vi "ecg_ncs_v4.vi"() -> ()   [LabVIEW 2016]
uses:
  <instrlib>/niUSRP/niUSRP Timestamp.ctl
  C:/Program Files/National Instruments/LabVIEW 2016/examples/Instrument IO/Serial/support/Serial - Settings.ctl
  State.ctl
  <vilib>/Instr/_visa.llb/VISA Configure Serial Port (Instr).vi
  <instrlib>/niUSRP/niUSRP Write Tx Data (2D CDB).vi
  <instrlib>/niUSRP/niUSRP Fetch Rx Data (2D CDB).vi
panel:
  in  "File Name 2":string="Test"
  in  "Path 2":path=path "D:/Research/SummerFall17Spring18/CnC/NCS/EcgNcsCorrelation/Labview Codes/ECG_NCS"
  out "#Loop = #Packets Received":i32
  out "ECGsample":i16
  out "PhNcs":dbl
  out "AmpNcs":dbl
  out "AmpNcsDS":dbl
  out "PhNcsDS":dbl
  out "error IO 2":errorcluster={"status"=FALSE, "code"=-1074118647, "source"=""}
  in  "Serial Settings":T1={"baud rate"=57600, "data bits"=8, "parity"=enum."None", "stop bits"=10, "flow control"=0} {"flow control" items=["None"=0, "XON/XOFF"=1, "RTS/CTS"=2, "DTR/DSR"=4]; "stop bits" items=["1.0"=10, "1.5"=15, "2.0"=20]; "data bits" min=5 max=8 step=1; "baud rate" items=["75"=75, "110"=110, "134"=134, "150"=150, "300"=300, "600"=600, "1200"=1200, "1800"=1800, "2400"=2400, "4800"=4800, "7200"=7200, "9600"=9600, "14400"=14400, "19200"=19200, "28800"=28800, "38400"=38400, "56000"=56000, "57600"=57600, "115200"=115200, "128000"=128000, "230400"=230400]}
  in  "VISA resource name":refnum<visa-resource-name>="bmd101"
  out "ECG":i16(graph)
  in  "byte count":u32=1
  out "Coerced Rx IQ Rate":dbl
  in  "Sampling Rate":i32=500
  out "Gain":dbl=-15.0
  out "Bandwidth":dbl=56000000.0
  out "Coerced Carrier Frequency":dbl=2000000000.0 format="%#.17g"
  out "Coerced Tx IQ rate":dbl=1000000.0
  out "error IO":errorcluster={"status"=FALSE, "code"=-1074118647, "source"=""}
  in  "Rx Number of Samples":i32=10000
  in  "Tab Control 2":enum32{"NI-294x/295x", "NI-2900/2901"}(tab)=enum."NI-2900/2901"
  in  "Rx carrier frequency [Hz]":dbl=2000000000.0 format="%#_6p"
  in  "Tx carrier frequency [Hz]":dbl=1000000000.0 format="%#_6p"
  in  "Start Trigger Time":T2={"whole seconds"=1, "fractional seconds"=0.0}
  in  "Tab Control":T3(tab)
  out "NCS tag Amp":dbl[](graph)=[0.011967714738528729, 0.012021355192189592, 0.012015275039596582, 0.011969166030167903, 0.011958890166168242, 0.012007893820858737, 0.012022893722444085, 0.011978222225113794, 0.011969989939463181, 0.012003099640895068]
  out "NCS tag Phase":dbl[](graph)=[0.011967714738528729, 0.012021355192189592, 0.012015275039596582, 0.011969166030167903, 0.011958890166168242, 0.012007893820858737, 0.012022893722444085, 0.011978222225113794, 0.011969989939463181, 0.012003099640895068]
  out "Tag Amp":dbl[](graph)
  out "Tag Phase":dbl[](graph)
  out "Tx Waveform Graph":waveform(dbl)[](graph)
  in  "Stop":bool
  in  "Channel 0\nTone Amplitude":dbl=0.707 step=0.05 format="%#.6g"
  in  "Channel 0 \nTone Frequency":dbl=5000.0 format="%#_6p"
  in  "Tx Waveform Size":dbl=2000.0
  in  "Device Name":refnum<k15>="MyB200"
  in  "Tx Gain":dbl=28.0 format="%#_6f"
  in  "Tx IQ Rate":dbl=1000000.0 format="%#_6p"
  in  "Rx Gain":dbl=32.0 format="%#_6f"
  in  "Rx IQ Rate":dbl=1000000.0 format="%#_6p"
  # "Rx Settings"
  # "Tx Settings"
  # "Note that on the NI-2900 and NI-2901, both Rx channels share an LO and both Tx channels share an LO. However, on the NI-294x/295x devices, Rx and Tx of channel 0 share an LO and Rx and Tx of channel 1 share an LO."
  # "Rx: Number of samples should be 1e6/512 in one loop."
  # "This Tx graph should always have end and start tied up since this is being sent in a loop continuously. Otherwise phase jumps will be noticed."
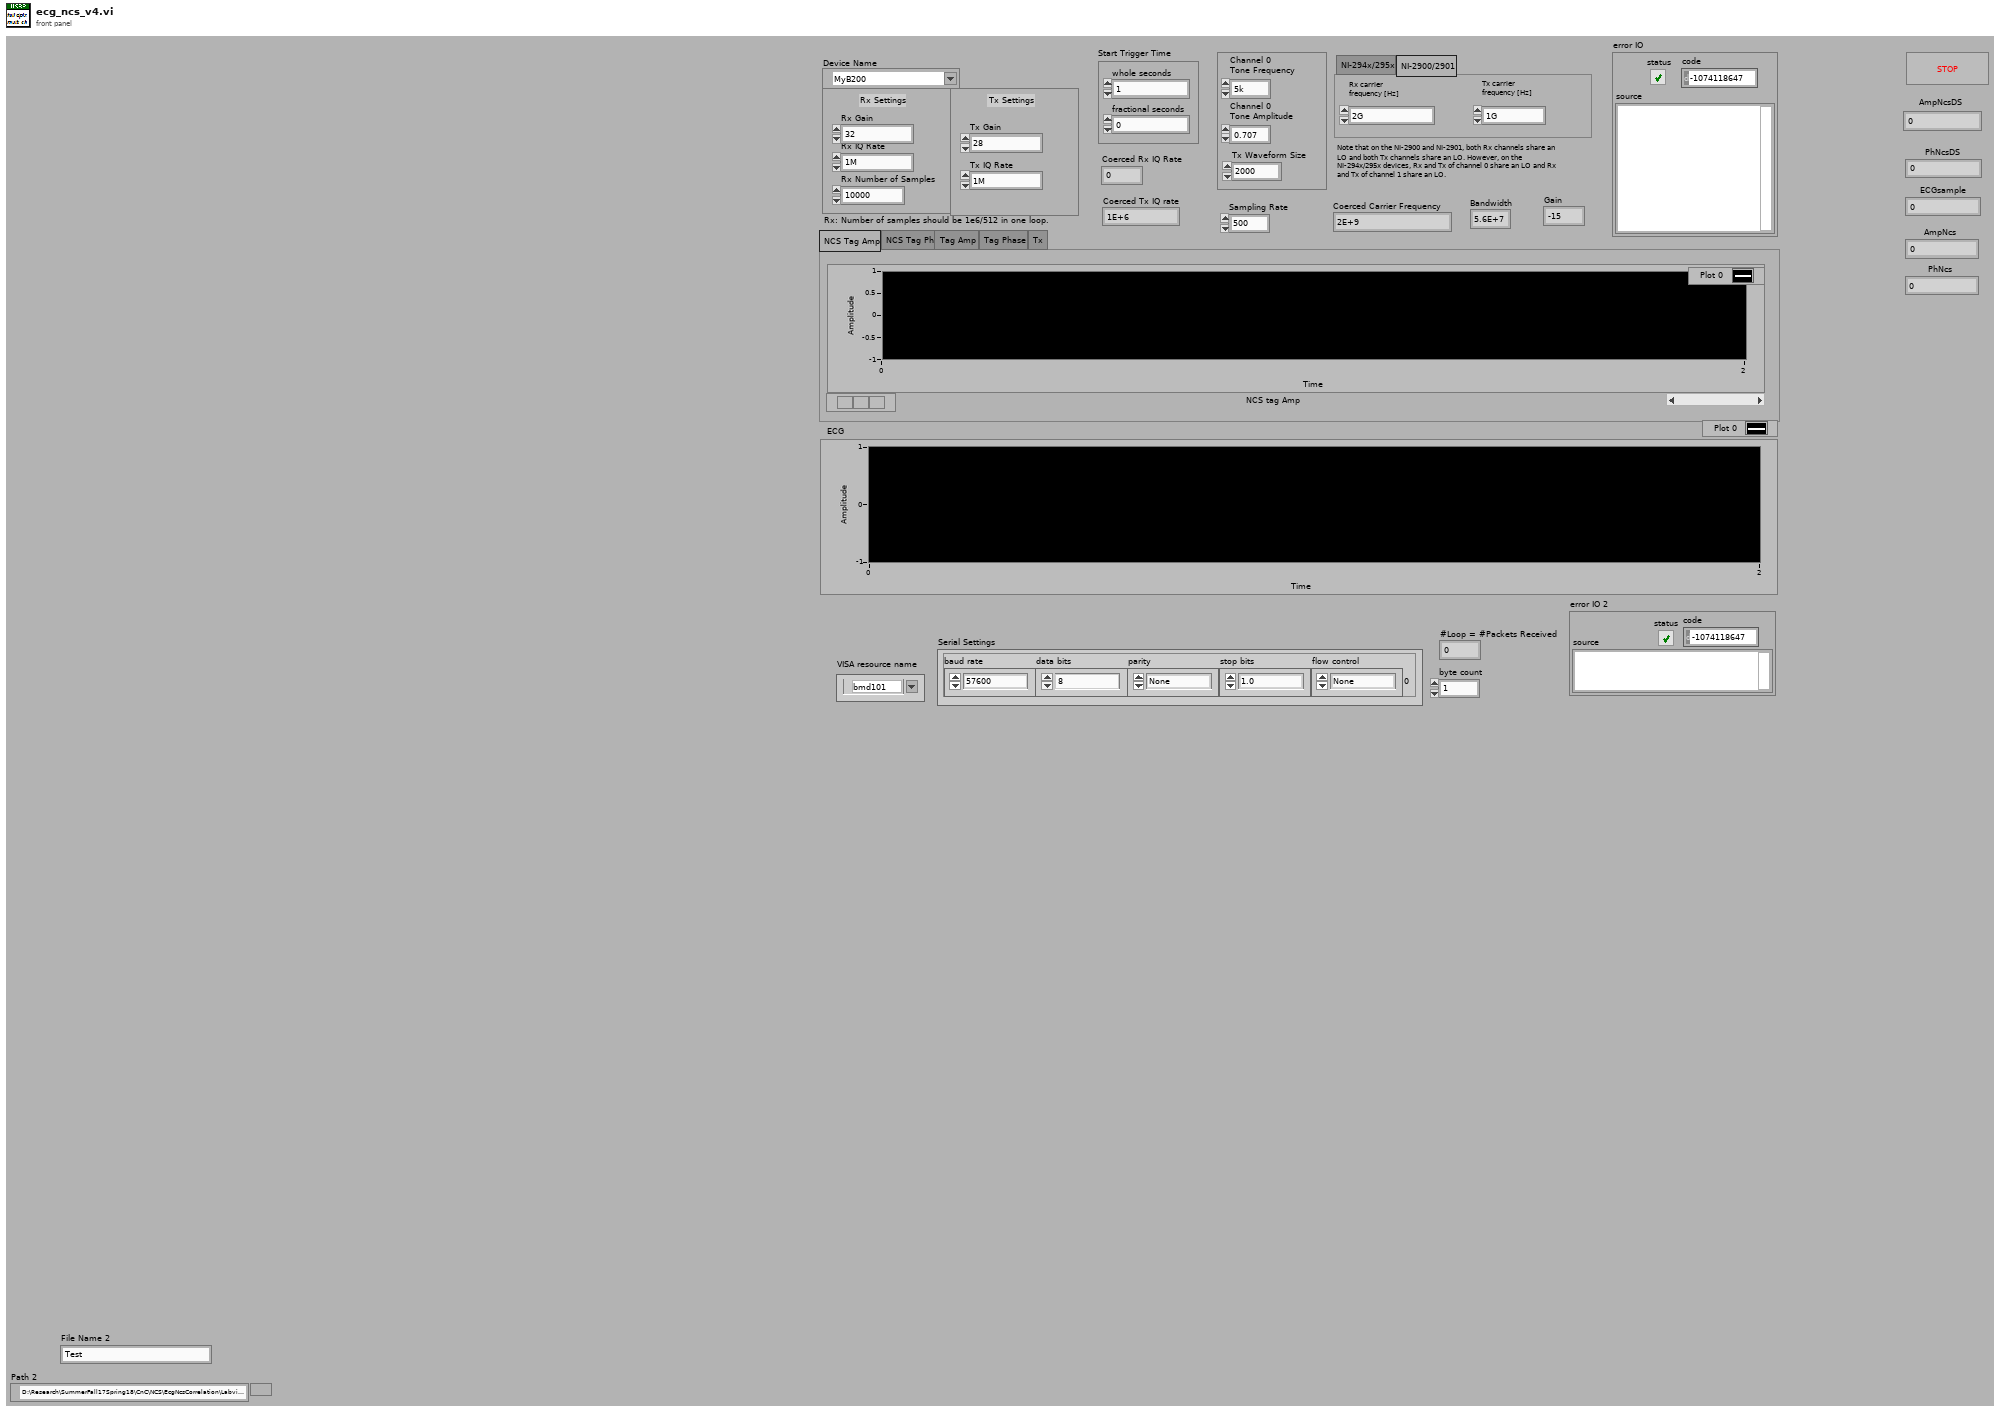
[diagram p1: front panel]
types:
  T1 = typedef "Serial - Settings.ctl" = cluster{"baud rate":u32, "data bits":u16, "parity":enum16{"None", "Odd", "Even", "Mark", "Space"}, "stop bits":u16, "flow control":u16}
  T2 = typedef "niUSRP Timestamp.ctl" = cluster{"whole seconds":u64, "fractional seconds":dbl}
  T3 = enum32{"NCS Tag Amp", "NCS Tag Ph", "Tag Amp", "Tag Phase", "Tx"}
  T4 = typedef "State.ctl" = enum16{"Initialize", "get byte", "check", "packet received", "packet approved"}
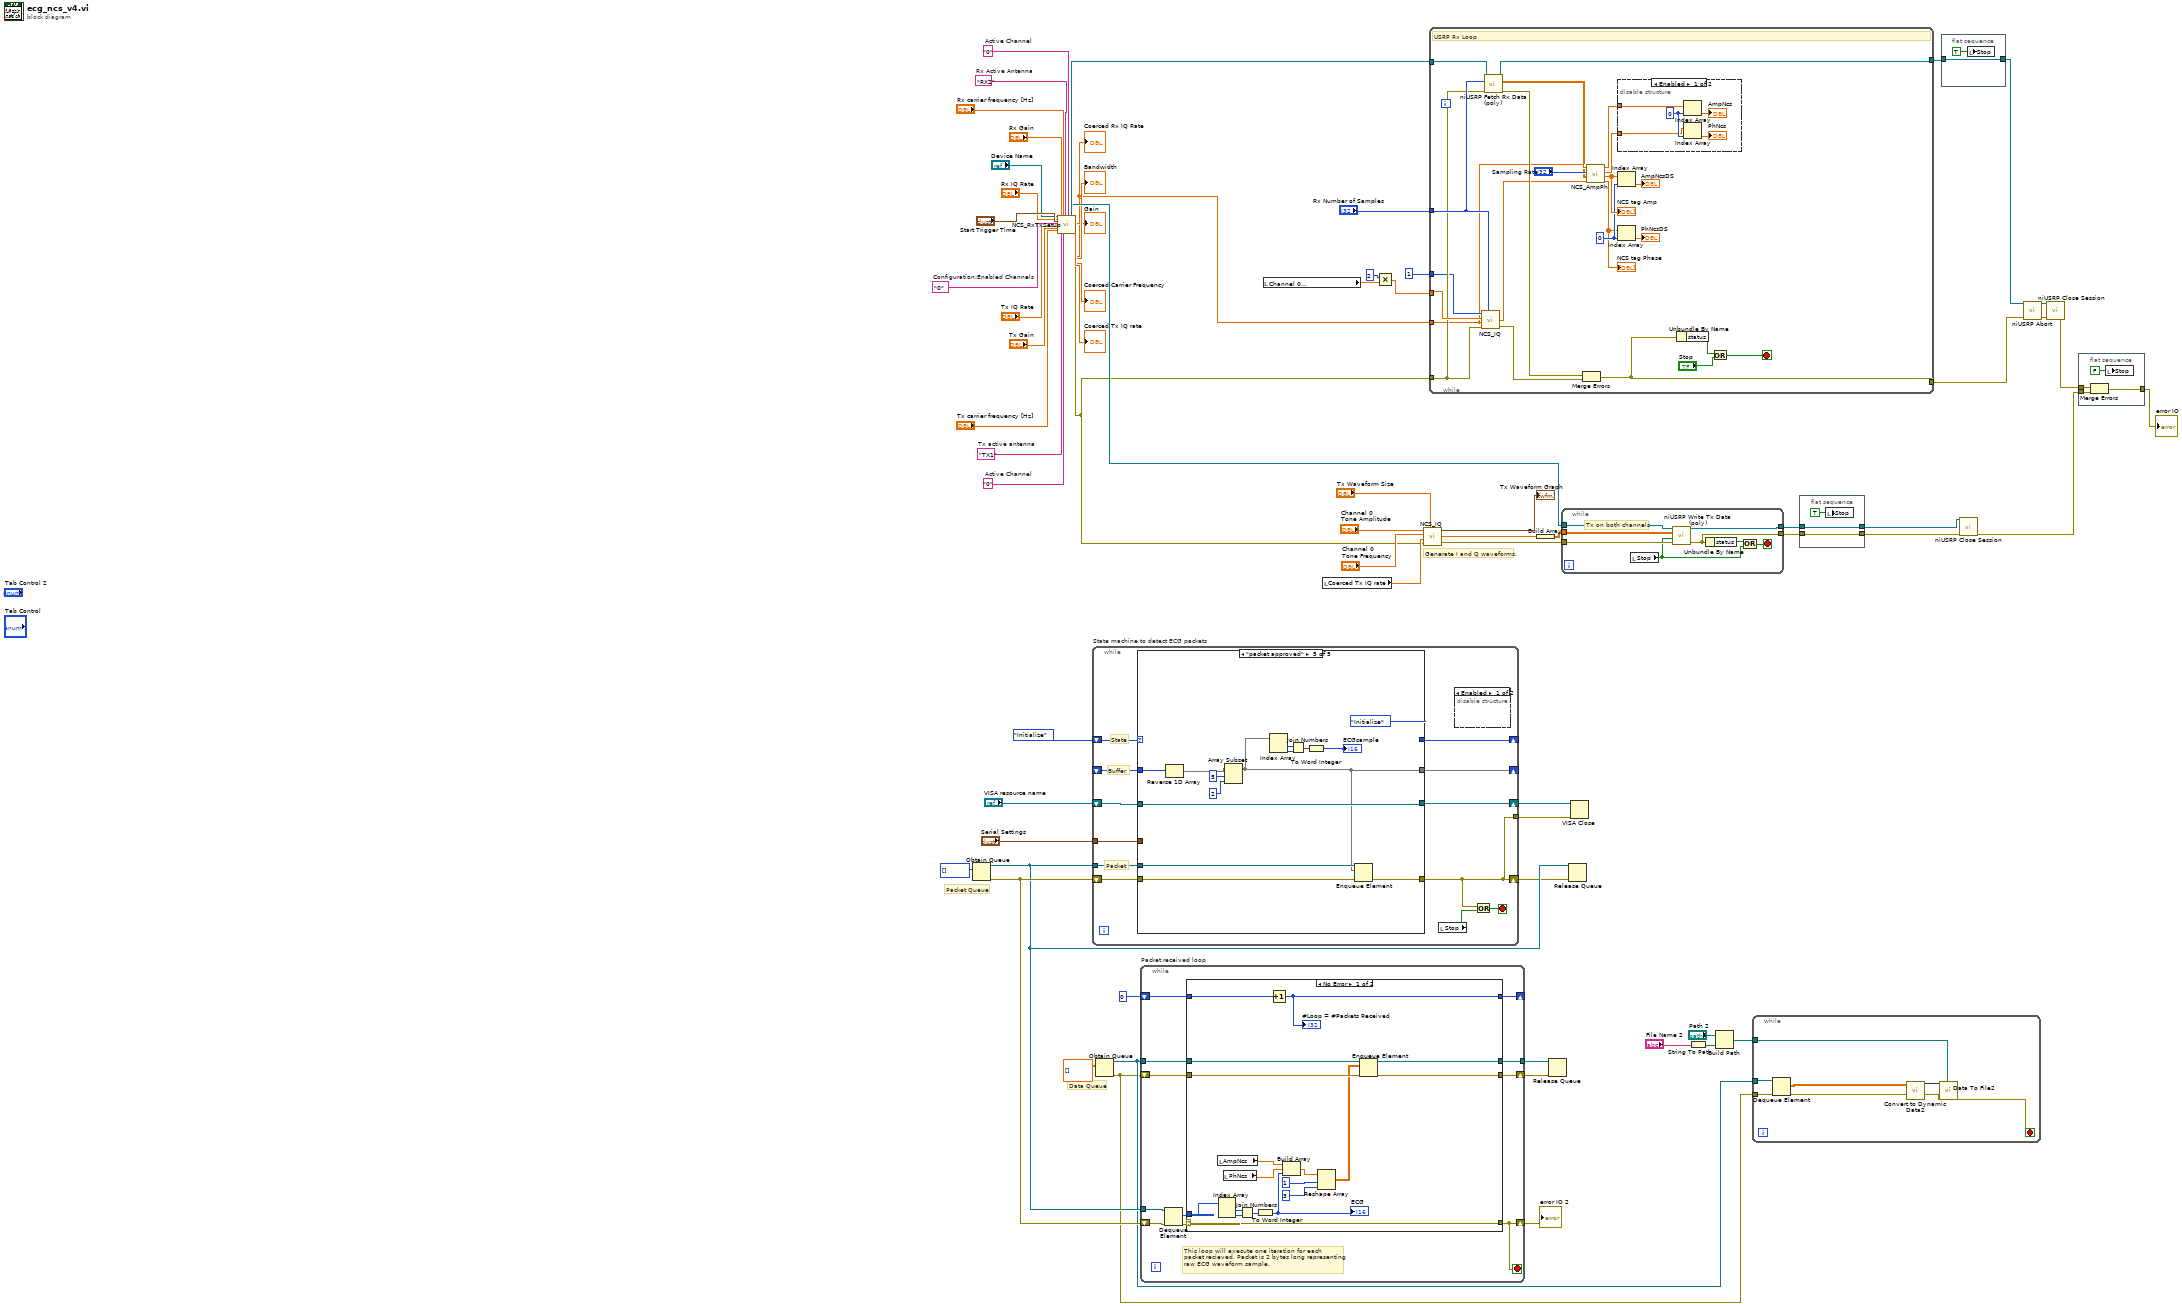
[diagram p0: block diagram]
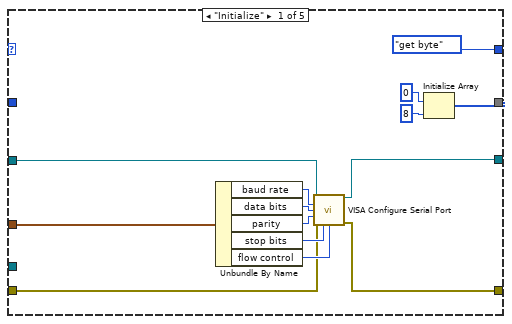
[diagram p4: hidden frame]
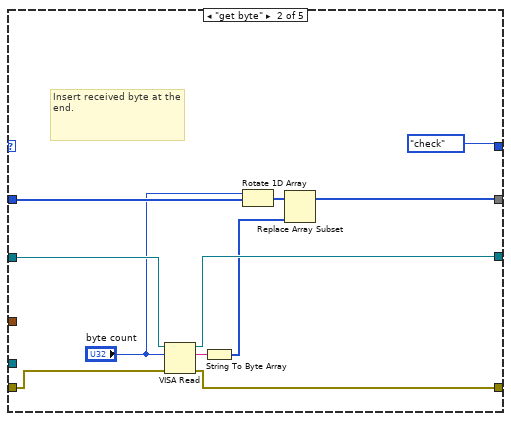
[diagram p5: hidden frame]
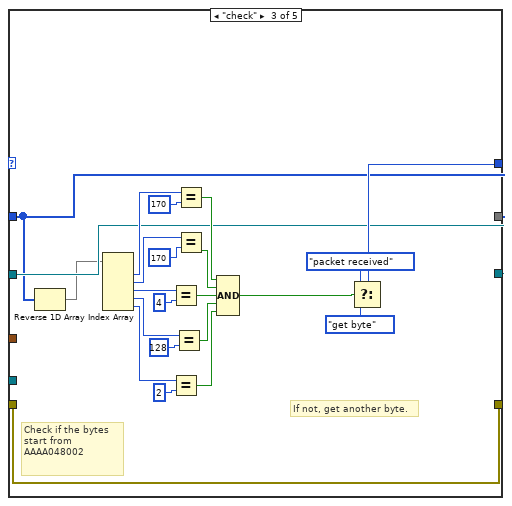
[diagram p6: hidden frame]
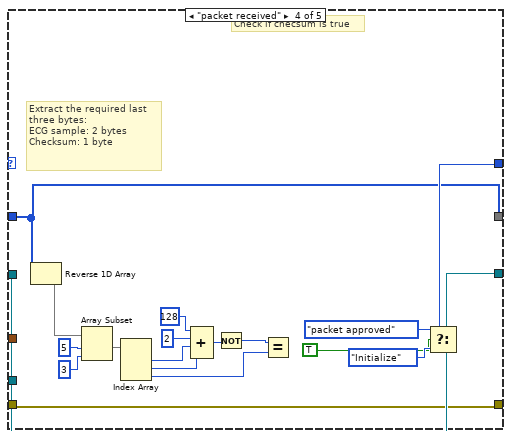
[diagram p7: hidden frame]
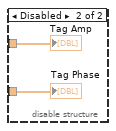
[diagram p8: hidden frame]
diagram:
  w22 = "0"  # Active Channel
  w23 = "0"  # Active Channel
  w58 = "RX2"  # Rx Active Antenna
  w54 = "TX1"  # Tx active antenna
  w40 = "0"  # Configuration:Enabled Channels
  # "Data Queue"
  # "Packet Queue"
  # "Generate I and Q waveforms."
  n1 = Obtain Queue(element data type=u8[] []) -> (queue out=w17:refnum<queue>, error out=w18:errorcluster)  [unwired: 4 in, 1 out]
  n2 = call "NCS_RxTxSetup.vi"("IVI Refnum in"="Device Name", "Rx IQ Rate"="Rx IQ Rate", "Start Trigger Time"="Start Trigger Time", "Configuration:Enabled Channels"=w40, "Tx IQ Rate"="Tx IQ Rate", "Tx Gain"="Tx Gain", "Tx carrier frequency [Hz]"="Tx carrier frequency [Hz]", "Rx Gain"="Rx Gain", "Tx active antenna"=w54, "Rx carrier frequency [Hz]"="Rx carrier frequency [Hz]", "Active Channel"=w22, "Rx Active Antenna"=w58, "Active Channel 2"=w23) -> ("session handle out"=w65:refnum<k15>, "IVI Refnum out"=w66:refnum<k15>, "Coerced Rx IQ Rate"=w21:dbl, "Bandwidth"=→"Bandwidth":dbl, "Gain"=→"Gain":dbl, "Carrier Frequency"=→"Coerced Carrier Frequency":dbl, "IQ Rate 2"=→"Coerced Tx IQ rate":dbl, "error out"=w33:errorcluster)  [unwired: 7 in]
  "Coerced Rx IQ Rate" <- w21
  n3 = while "State machine to detect ECG packets" {
    shift-right: [w69] -> w12
    shift-left: w18 -> [w75]
    shift-right: [w78] -> _
    shift-left: State."Initialize" ("State") -> [w77]
    shift-right: [w74] -> _
    shift-left: _ -> [w76]
    tunnel: w17 -> [w73]
    shift-right: [w72] -> w13
    shift-left: "VISA resource name" -> [w71]
    tunnel: "Serial Settings" -> [w70]
    tunnel: [w69] -> w11
    stop <- w68 stop-if-true
    # "State"
    # "Buffer"
    # "Packet"
    n4 = case shown="\"packet approved\"" w77 {
      tunnel: [w89 w101 w105 w128 w147] -> w74
      tunnel: [State."get byte" ("State") State."check" ("f") w125 w134 State."Initialize" ("State")] -> w78
      tunnel: w76 -> [_ w94 w105 w128 w151]
      tunnel: w75 -> [w83 w98 w126 w135 w154]
      tunnel: [w82 w97 w126 w135 w153] -> w69
      tunnel: w73 -> [_ _ _ _ w155]
      tunnel: [w81 w99 w106 w142 w152] -> w72
      tunnel: w71 -> [w80 w100 w106 w142 w152]
      tunnel: w70 -> [w79 _ _ _ _]
      frame "Initialize" {
        n5 = Unbundle By Name(w79) -> ("baud rate"=w88:u32, "data bits"=w87:u16, "parity"=w86:enum16{"None", "Odd", "Even", "Mark", "Space"}, "stop bits"=w85:u16, "flow control"=w84:u16)
        n6 = call-poly "VISA Configure Serial Port"("VISA resource name"=w80, "baud rate (9600)"=w88, "data bits (8)"=w87, "parity (0:none)"=w86, "error in (no error)"=w83, "stop bits (10: 1 bit)"=w85, "flow control (0:none)"=w84) -> ("VISA resource name out"=w81:refnum<visa-resource-name>, "error out"=w82:errorcluster)  [unwired: 3 in, 4 out]
        n7 = Initialize Array(u8 0, 8 ("dimension size")) -> (w89:u8[])
      }
      frame "get byte" {
        # "Insert received byte at the end."
        n8 = VISA Read(VISA resource name=w100, byte count="byte count", error in (no error)=w98) -> (VISA resource name out=w99:refnum<visa-resource-name>, read buffer=w96:string, error out=w97:errorcluster)  [unwired: 1 out]
        n9 = String To Byte Array(string=w96) -> (unsigned byte array=w95:u8[])
        n10 = Rotate 1D Array(1:w94, 2:"byte count") -> (0:w102:u8[])
        n11 = Replace Array Subset(array=w102, new element=w95) -> (w101:u8[])  [unwired: 1 in]
      }
      frame "check" {
        # "If not, get another byte."
        # "Check if the bytes start from AAAA048002"
        n12 = Reverse 1D Array(array=w105) -> (reversed array=w104:u8[])
        n13 = Index Array(array=w104) -> (element #1=w112:u8, element #2=w111:u8, element #3=w110:u8, element #4=w109:u8, element #5=w108:u8)  [unwired: 5 in]
        n14 = Equal?(x=w110, y=u8 4 ("element")) -> (x = y?=w115:bool)
        n15 = Equal?(x=w108, y=u8 2 ("element")) -> (x = y?=w113:bool)
        n16 = Equal?(x=w109, y=u8 128 ("element")) -> (x = y?=w114:bool)
        n17 = Equal?(x=w112, y=u8 170 ("element")) -> (x = y?=w117:bool)
        n18 = Equal?(x=w111, y=u8 170 ("element")) -> (x = y?=w116:bool)
        n19 = Compound Arithmetic op=AND(w117, w116, w115, w114, w113) -> (w107:bool)
        n20 = Select(t=State."packet received" ("f"), s=w107, f=State."get byte") -> (s? t:f=w125:T4)
      }
      frame "packet received" {
        # "Check if checsum is true"
        # "Extract the required last three bytes: \nECG sample: 2 bytes\nChecksum: 1 byte"
        n21 = Reverse 1D Array(array=w128) -> (reversed array=w127:u8[])
        n22 = Array Subset(array=w127, index=5, length=3 ("index")) -> (w141:u8[])
        n23 = Index Array(array=w141) -> (element #1=w136:u8, element #2=w137:u8, element #3=w138:u8)  [unwired: 3 in]
        n24 = Compound Arithmetic op=ADD(u8 128 ("element"), u8 2 ("element"), w136, w137) -> (w131:u8)
        n25 = Not(x=w131) -> (.not. x?=w130:u8)
        n26 = Equal?(x=w130, y=w138) -> ()  [unwired: 1 out]
        n27 = Select(t=State."packet approved" ("State"), s=TRUE, f=State."Initialize" ("State")) -> (s? t:f=w134:T4)
      }
      frame "packet approved" {
        n28 = Reverse 1D Array(array=w151) -> (reversed array=w150:u8[])
        n29 = Array Subset(array=w150, index=5, length=2 ("index")) -> (w147:u8[])
        n30 = Index Array(array=w147) -> (element #1=w146:u8, element #2=w148:u8)  [unwired: 2 in]
        n31 = Join Numbers(hi=w146, lo=w148) -> ((hi.lo)=w149:u16)
        n32 = To Word Integer(number=w149) -> (16bit integer=→"ECGsample":i16)
        n33 = Enqueue Element(queue=w155, element=w147, error in (no error)=w154) -> (error out=w153:errorcluster)  [unwired: 1 in, 2 out]
      }
    }
    n34 = local read "Stop"() -> (w67:bool)
    n35 = disable-structure shown="Enabled" {
      frame Enabled {
      }
      frame Disabled {
      }
    }
    n36 = Or(x=w69, y=w67) -> (x .or. y?=w68:bool)
  }
  n37 = Obtain Queue(element data type=dbl[][] []) -> (queue out=w3:refnum<queue>, error out=w2:errorcluster)  [unwired: 4 in, 1 out]
  n38 = while "Packet received loop" {
    shift-right: [w165] -> w14
    shift-left: w18 -> [w169]
    tunnel: w17 -> [w168]
    shift-right: [w163] -> _
    shift-left: 0 -> [w164]
    tunnel: w3 -> [w162]
    tunnel: [w160] -> w5
    shift-right: [w159] -> w1
    shift-left: w2 -> [w161]
    stop <- w165 stop-if-true
    # "This loop will execute one iteration for each\npacket recieved. Packet is 2 bytes long representing \nraw ECG waveform sample."
    n39 = Dequeue Element(queue=w168, error in (no error)=w169) -> (element=w167:u8[], error out=w166:errorcluster)  [unwired: 1 in, 2 out]
    n40 = case shown="No Error" w166 {
      selector: w166 -> [w175 w191]
      tunnel: w167 -> [w187 _]
      tunnel: [w175 w191] -> w165
      tunnel: w164 -> [w183 w190]
      tunnel: [w182 w190] -> w163
      tunnel: w162 -> [w174 w189]
      tunnel: w161 -> [w173 w188]
      tunnel: [w171 w188] -> w159
      tunnel: [w170 w189] -> w160
      frame No Error {
        n41 = local read "AmpNcs"() -> (w177:dbl)
        n42 = Index Array(array=w187) -> (element #1=w186:u8, element #2=w185:u8)  [unwired: 2 in]
        n43 = local read "PhNcs"() -> (w176:dbl)
        n44 = Join Numbers(hi=w186, lo=w185) -> ((hi.lo)=w184:u16)
        n45 = To Word Integer(number=w184) -> (16bit integer=w178:i16)
        "ECG" <- w178
        n46 = Increment(x=w183) -> (x+1=w182:i32)
        "#Loop = #Packets Received" <- w182
        n47 = Build Array(w177, w176, w178) -> (w181:dbl[])
        n48 = Reshape Array(w181, 1 ("dimension size"), 3 ("dimension size")) -> (w172:dbl[][])
        n49 = Enqueue Element(queue=w174, element=w172, error in (no error)=w173) -> (queue out=w170:refnum<queue>, error out=w171:errorcluster)  [unwired: 1 in, 1 out]
      }
      frame Error {
      }
    }
  }
  "error IO 2" <- w14
  n50 = local read "Channel 0 \nTone Frequency"() -> (w39:dbl)
  n51 = local read "Coerced Tx IQ rate"() -> (w34:dbl)
  n52 = Multiply(x=2, y=w39) -> (x*y=w38:dbl)
  n53 = call "NCS_IQ.vi"("Tone Amplitude"="Channel 0\nTone Amplitude", "Waveform Size"="Tx Waveform Size", "Tone Frequency"="Channel 0 \nTone Frequency", "Coerced IQ rate"=w34, "error in (no error)"=w33) -> ("IQ waveform"=→"Tx Waveform Graph":waveform(dbl)[], "IQ waveform array"=w31:cdb[], "error out"=w32:errorcluster)  [unwired: 1 in]
  n54 = while {
    tunnel: w66 -> [w214]
    tunnel: w33 -> [w207]
    tunnel: [w213] -> w50
    tunnel: "Rx Number of Samples" -> [w209]
    tunnel: w21 -> [w203]
    tunnel: [w204] -> w42
    tunnel: w38 -> [w208]
    tunnel: 1 -> [w205]
    stop <- w210 stop-if-true
    w195 = 0
    # "USRP Rx Loop"
    n55 = call "NCS_IQ.vi"("Tone Amplitude"=w205, "Waveform Size"=w209, "Tone Frequency"=w208, "Coerced IQ rate"=w203, "error in (no error)"=w207) -> ("IQ waveform array"=w200:cdb[], "error out"=w206:errorcluster)  [unwired: 1 in, 1 out]
    n56 = call-poly <instrlib>:"niUSRP Fetch Rx Data (poly).vi"("session handle"=w214, "number of samples"=w209, "error in (no error)"=w207) -> ("session handle out"=w213:refnum<k15>, "data"=w201:cdb[][], "error out"=w211:errorcluster)  [unwired: 9 in, 1 out]
    n57 = Merge Errors(w211, w206) -> (w204:errorcluster)
    n58 = call "NCS_AmpPh.vi"("IQ"=w200, "data"=w201, "Sampling Rate"="Sampling Rate", "Coerced Rx IQ Rate"=w203) -> ("Phase DownSampled"=w194:dbl[], "Amp DownSampled"=w196:dbl[], "Phase"=w198:dbl[], "Amplitude"=w199:dbl[])  [unwired: 4 in]
    "NCS tag Amp" <- w196
    "NCS tag Phase" <- w194
    n59 = disable-structure shown="Enabled" {
      disable-tunnel: w199 -> [w218 w221]
      disable-tunnel: w198 -> [w217 w220]
      frame Enabled {
        w219 = 0
        n60 = Index Array(array=w218, index=w219) -> (element=→"AmpNcs":dbl)
        n61 = Index Array(array=w217, index=w219) -> (element=→"PhNcs":dbl)
      }
      frame Disabled {
        "Tag Amp" <- w221
        "Tag Phase" <- w220
      }
    }
    n62 = Index Array(array=w196, index=w195) -> (element=→"AmpNcsDS":dbl)
    n63 = Index Array(array=w194, index=w195) -> (element=→"PhNcsDS":dbl)
    n64 = Unbundle By Name(w204) -> ("status"=w212:bool)
    n65 = Or(x=w212, y="Stop") -> (x .or. y?=w210:bool)
  }
  n66 = Build Array(w31) -> (w62:cdb[][])
  n67 = Release Queue(queue=w5, error in (no error)=w1) -> ()  [unwired: 1 in, 3 out]
  n68 = while {
    tunnel: w65 -> [w229]
    tunnel: w32 -> [w228]
    tunnel: [w226] -> w53
    tunnel: [w224] -> w48
    tunnel: w62 -> [w222]
    stop <- w225 stop-if-true
    # "Tx on both channels"
    n69 = local read "Stop"() -> (w223:bool)
    n70 = call-poly <instrlib>:"niUSRP Write Tx Data (poly).vi"("session handle"=w229, "data"=w222, "end of data?"=w223, "error in (no error)"=w228) -> ("session handle out"=w224:refnum<k15>, "error out"=w226:errorcluster)  [unwired: 10 in]
    n71 = Unbundle By Name(w226) -> ("status"=w227:bool)
    n72 = Compound Arithmetic op=OR(w227, w223) -> (w225:bool)
  }
  n73 = Release Queue(queue=w17, error in (no error)=w12) -> ()  [unwired: 1 in, 3 out]
  n74 = VISA Close(VISA resource name=w13, error in (no error)=w11) -> ()  [unwired: 1 out]
  n75 = String To Path(string="File Name 2") -> (path=w9:path)
  n76 = Build Path(base path="Path 2", name or relative path=w9) -> (appended path=w4:path)
  n77 = while {
    tunnel: w4 -> [w235]
    tunnel: w3 -> [w234]
    tunnel: w2 -> [w233]
    stop <- w230 stop-if-true
    n78 = Dequeue Element(queue=w234, error in (no error)=w233) -> (element=w232:dbl[][], error out=w231:errorcluster)  [unwired: 1 in, 2 out]
    n79 = call "Convert to Dynamic Data2"("2D Array"=w232) -> ("Dynamic Data Type"=w236:dynamicdata)  [unwired: 3 in]
    n80 = call "Data To File2"("Signals"=w236, "error in (no error)"=w231, "Filename"=w235) -> ("error out"=w230:errorcluster)  [unwired: 14 in, 2 out]
  }
  n81 = flat-sequence {
    tunnel: [w238] -> w52
    tunnel: w53 -> [w238]
    tunnel: [w237] -> w49
    tunnel: w48 -> [w237]
    frame #0 {
      n82 = local write "Stop"(TRUE ("STOP")) -> ()
    }
  }
  n83 = flat-sequence {
    tunnel: [w240] -> w51
    tunnel: w50 -> [w240]
    frame #0 {
      n84 = local write "Stop"(TRUE ("STOP")) -> ()
    }
  }
  n85 = call <instrlib>:"niUSRP Close Session.vi"("session handle"=w49, "error in (no error)"=w52) -> ("error out"=w47:errorcluster)  [unwired: 13 in]
  n86 = call <instrlib>:"niUSRP Abort.vi"("session handle"=w51, "error in (no error)"=w42) -> ("session handle out"=w64:refnum<k15>, "error out"=w63:errorcluster)  [unwired: 12 in]
  n87 = call <instrlib>:"niUSRP Close Session.vi"("session handle"=w64, "error in (no error)"=w63) -> ("error out"=w44:errorcluster)  [unwired: 13 in]
  n88 = flat-sequence {
    tunnel: w47 -> [w244]
    tunnel: [w243] -> w45
    tunnel: w44 -> [w242]
    frame #0 {
      n89 = Merge Errors(w242, w244) -> (w243:errorcluster)
      n90 = local write "Stop"(FALSE ("STOP")) -> ()
    }
  }
  "error IO" <- w45
